vi "CRYPEAQ log2.vi"(11 "a":dbl=1.0) -> (3 "log2":dbl)   [LabVIEW 2013]
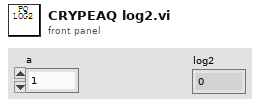
[diagram p1: front panel]
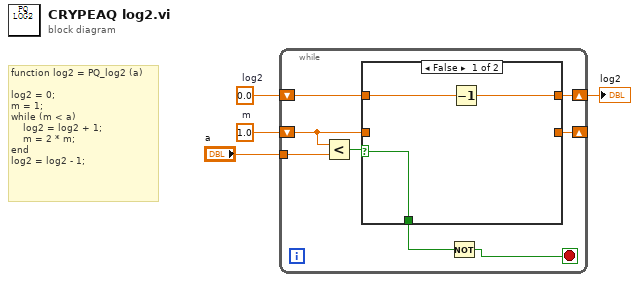
[diagram p0: block diagram]
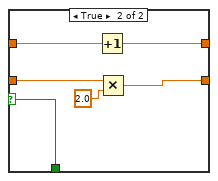
[diagram p2: hidden frame]
diagram:
  w3 = 0.0  # log2
  w4 = 1.0  # m
  # "function log2 = PQ_log2 (a)\n\nlog2 = 0;\nm = 1;\nwhile (m < a)\n    log2 = log2 + 1;\n    m = 2 * m;\nend\nlog2 = log2 - 1;"
  n1 = while {
    tunnel: "a" -> [w11]
    shift-right: [w9] -> w1
    shift-left: w3 -> [w10]
    shift-right: [w6] -> _
    shift-left: w4 -> [w7]
    stop <- w5 stop-if-true
    n2 = Less?(x=w7, y=w11) -> (x < y?=w12:bool)
    n3 = case shown="False" w12 {
      selector: w12 -> [w15 w19]
      tunnel: w10 -> [w14 w21]
      tunnel: [w13 w20] -> w9
      tunnel: [w15 w19] -> w8
      tunnel: w7 -> [_ w18]
      tunnel: [_ w17] -> w6
      frame False {
        n4 = Decrement(x=w14) -> (x-1=w13:dbl)
      }
      frame True {
        n5 = Increment(x=w21) -> (x+1=w20:dbl)
        n6 = Multiply(x=w18, y=2.0) -> (x*y=w17:dbl)
      }
    }
    n7 = Not(x=w8) -> (.not. x?=w5:bool)
  }
  "log2" <- w1
